vi "Test_WriteValue_CheckTerminal_TerminalUpdated.vi"(8 "error in (no error)":errorcluster, 11 "TestCase in":refnum<class "TestTerminalValueBinding.lvclass">) -> (0 "error out":errorcluster, 3 "TestCase out":refnum<class "TestTerminalValueBinding.lvclass">)   [LabVIEW 2017, in "TestTerminalValueBinding.lvclass"]
uses:
  TestTerminalValueBinding.lvclass
  Source/Concrete/TerminalValueBinding/TerminalValueBinding.lvclass
  C:/Git/composed-transport/Source/ITransport/ITransport.lvclass
  Source/ITransport/ITransport.lvclass
panel:
  in  "Numeric":i32
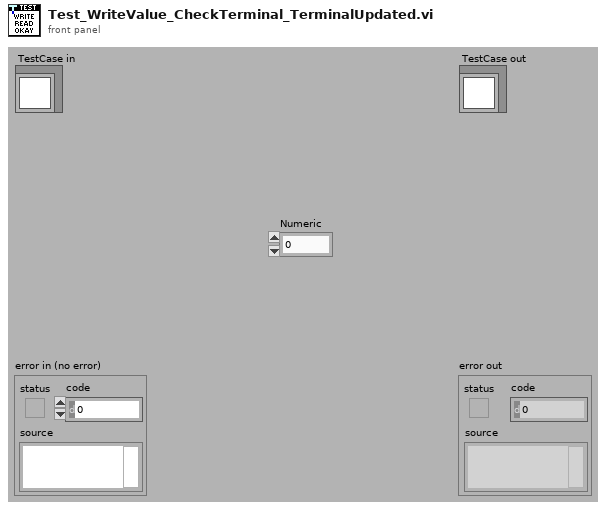
[diagram p1: front panel]
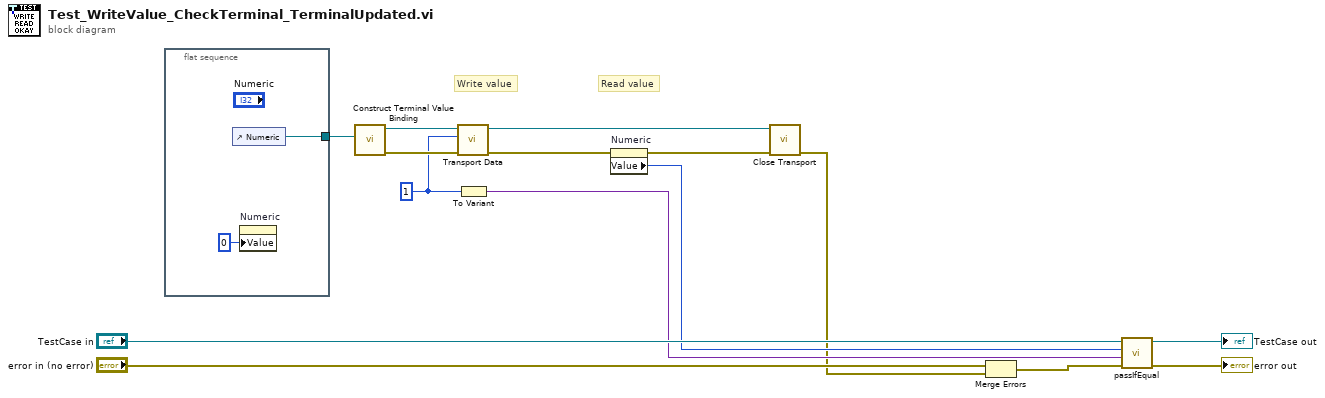
[diagram p0: block diagram]
diagram:
  w8 = 1
  # "Read value"
  # "Write value"
  n1 = flat-sequence {
    tunnel: [w17] -> w5
    frame #0 {
      n2 = control-ref of="Numeric"() -> (w17:refnum<vi>)
      n3 = property on="Numeric" class="DigNum (strict)"("Value"=0 ("Numeric")) -> ()  [unwired: 2 in, 2 out]
    }
  }
  n4 = call "Construct Terminal Value Binding.vi"("Ctl Refnum"=w5) -> ("error out"=w9:errorcluster, "TerminalValueBinding Out"=w11:refnum<class "TerminalValueBinding.lvclass">)  [unwired: 9 in]
  n5 = call "Transport Data.vi"("error in (no error)"=w9, "Value"=w8, "ITransport in"=w11) -> ("error out"=w4:errorcluster, "ITransport out"=w6:refnum<class "TerminalValueBinding.lvclass">)  [unwired: 7 in]
  n6 = To Variant(anything=w8) -> (Variant=w7:variant)
  n7 = property on="Numeric" class="DigNum (strict)"(error in=w4) -> (error out=w3:errorcluster, "Value"=w2:i32)  [unwired: 1 in, 1 out]
  n8 = call-dynamic "Close Transport.vi"("error in (no error)"=w3, "ITransport in"=w6) -> ("error out"=w1:errorcluster)  [unwired: 9 in]
  n9 = Merge Errors("error in (no error)", w1) -> (w10:errorcluster)
  n10 = call-dynamic "passIfEqual.vi"("error in (no error)"=w10, "y"=w7, "x"=w2, "TestCase in"="TestCase in") -> ("error out"=→"error out":errorcluster, "TestCase out"=→"TestCase out":refnum<class "TestTerminalValueBinding.lvclass">)  [unwired: 6 in]
